vi "CurrentTrace.vi"() -> ()   [LabVIEW 2009]
uses:
  <vilib>/Utility/file.llb/Write To Spreadsheet File (DBL).vi
  <vilib>/express/express analysis/Spectral/XNode/ExpressSpectralMeasurementsBlockNode.xnode
  <vilib>/express/express analysis/Spectral/Block/exnSpectralBlock spectral measurements peak poly.vi
  <vilib>/express/express analysis/Spectral/Block/exnSpectralBlock spectral measurements peak DDT.vi
panel:
  in  "Enable":bool=TRUE
  in  "Filename":path=path "test.tdms"
  in  "String":string
  in  "Save Filtered Spectrum":bool
  in  "file path (use dialog) 4":path
  in  "Save Filtered Waveform":bool
  in  "file path (use dialog) 3":path
  in  "Save Unfiltered Spectrum":bool
  in  "file path (use dialog) 2":path
  in  "Save Unfiltered Waveform":bool
  in  "Boolean":bool
  in  "Bandpass Upper Cut-Off":dbl=313000.0 caption="Upper Cut-Off"
  in  "Bandpass Lower Cut-Off":dbl=312000.0 caption="Lower Cut-Off"
  in  "Low-Pass Cut-Off (Hz)":dbl=10000.0 caption="Lower Cut-Off"
  out "Filtered Spectrum":dynamicdata(graph)
  out "Unfiltered Spectrum":dynamicdata(graph)
  out "Filtered Signal":dynamicdata(graph)
  out "Unfiltered Signal":dynamicdata(graph)
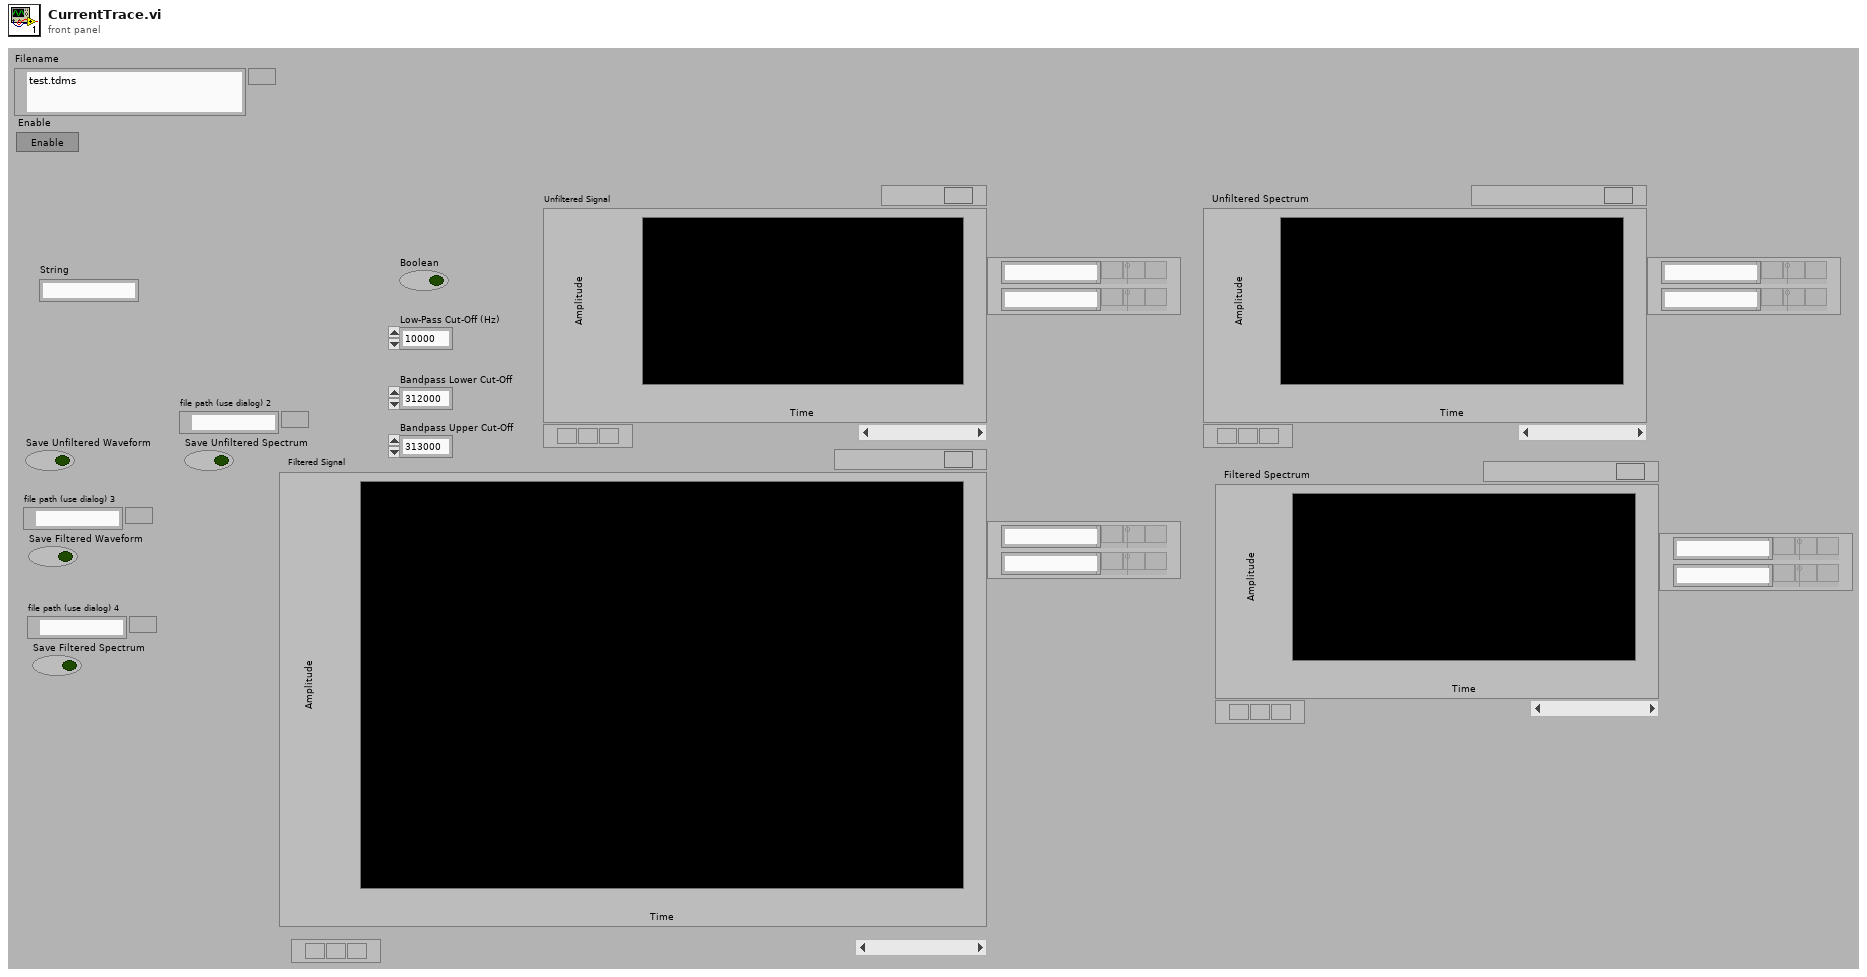
[diagram p1: front panel]
types:
  T1 = enum16{"open", "replace", "create", "open or create", "replace or create", "replace or create with confirmation"}
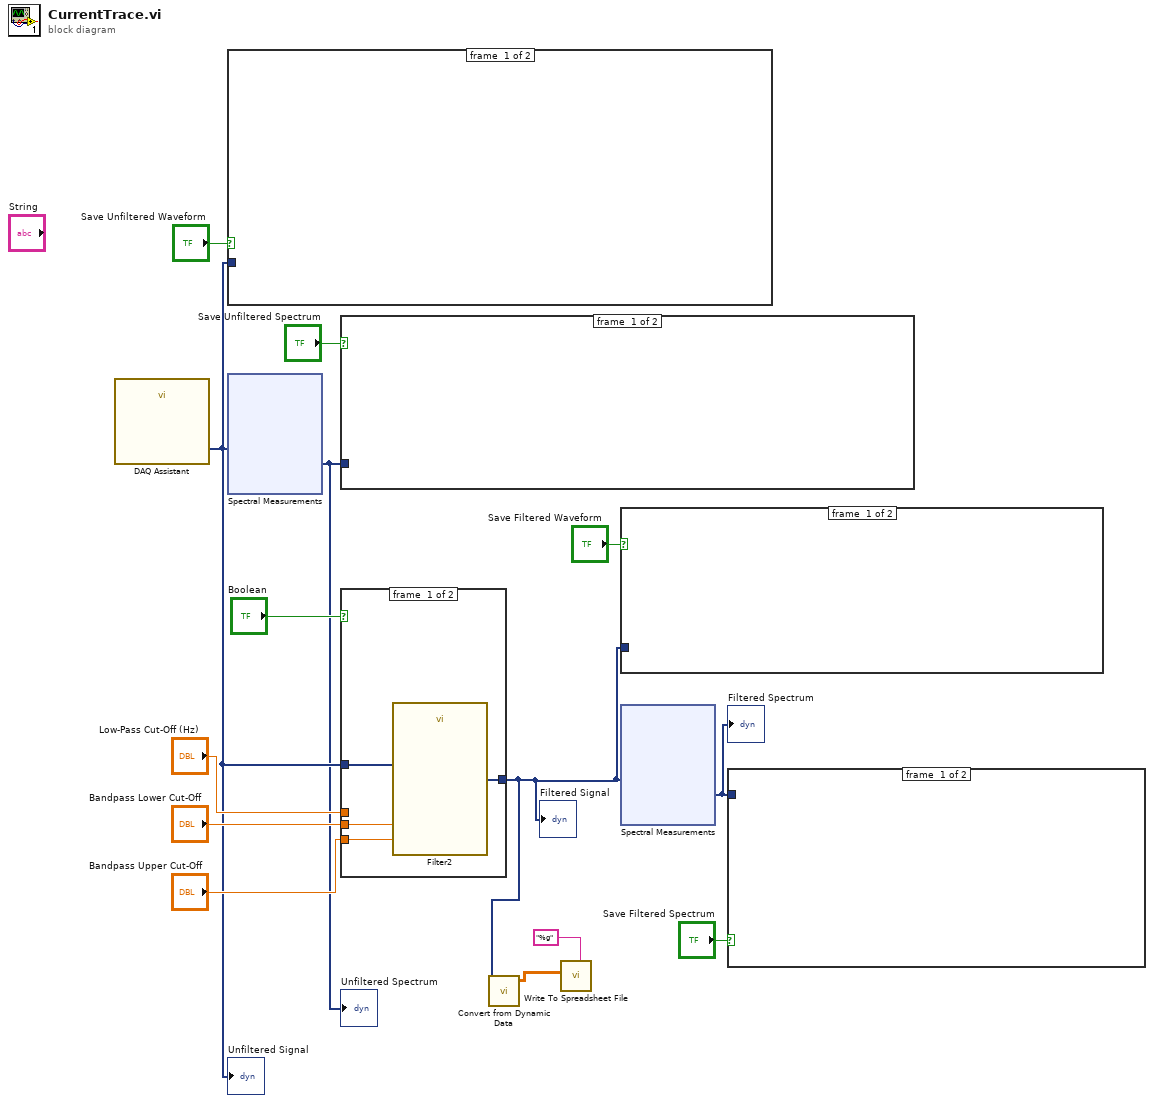
[diagram p0: block diagram]
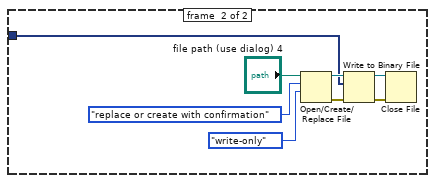
[diagram p2: hidden frame]
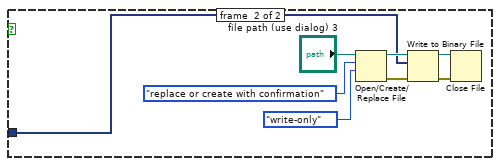
[diagram p3: hidden frame]
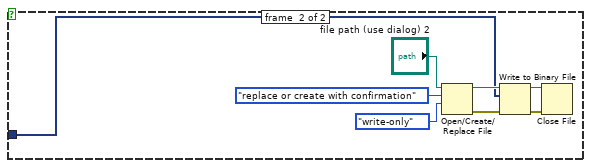
[diagram p4: hidden frame]
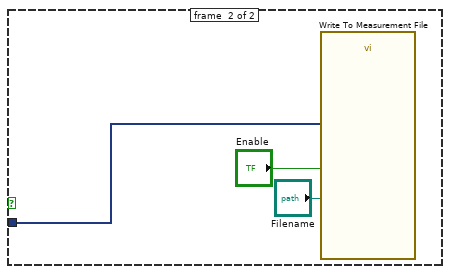
[diagram p5: hidden frame]
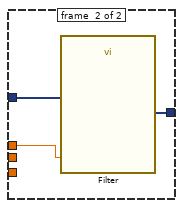
[diagram p6: hidden frame]
diagram:
  n1 = call "DAQ Assistant"() -> ("data"=w10:dynamicdata)  [unwired: 17 in, 2 out]
  "Unfiltered Signal" <- w10
  n2 = case shown="True" "Save Unfiltered Waveform" {
    tunnel: w10 -> [_ w17]
    frame #0 {
    }
    frame #1 {
      n3 = call "Write To Measurement File"("Signals"=w17, "Enable"="Enable", "Filename"="Filename") -> ()  [unwired: 14 in, 3 out]
    }
  }
  n4 = xnode "Spectral Measurements"("Signals"=w10) -> ("FFT - (Peak)"=w7:dynamicdata)  [unwired: 1 in, 2 out]
  "Unfiltered Spectrum" <- w7
  n5 = case shown="True" "Save Unfiltered Spectrum" {
    tunnel: w7 -> [_ w18]
    frame #0 {
    }
    frame #1 {
      n6 = Open/Create/Replace File(file path (use dialog)="file path (use dialog) 2", operation (0:open)=T1."replace or create with confirmation", access (0:read/write)=enum16{"read/write", "read-only", "write-only"}."write-only") -> (refnum out=w22:refnum<file>, error out=w21:errorcluster)  [unwired: 3 in, 1 out]
      n7 = Write to Binary File(file (use dialog)=w22, data=w18, error in=w21) -> (refnum out=w20:refnum<file>, error out=w19:errorcluster)  [unwired: 3 in, 1 out]
      n8 = Close File(refnum=w20, error in=w19) -> ()  [unwired: 2 out]
    }
  }
  n9 = case shown="True" "Boolean" {
    tunnel: "Low-Pass Cut-Off (Hz)" -> [_ w31]
    tunnel: "Bandpass Lower Cut-Off" -> [w29 _]
    tunnel: "Bandpass Upper Cut-Off" -> [w28 _]
    tunnel: w10 -> [w27 w32]
    tunnel: [w26 w30] -> w3
    frame #0 {
      n10 = call "Filter2"("Lower Cut-Off"=w29, "Upper Cut-Off"=w28, "Signal"=w27) -> ("Filtered Signal"=w26:dynamicdata)  [unwired: 7 in, 1 out]
    }
    frame #1 {
      n11 = call "Filter"("Lower Cut-Off"=w31, "Signal"=w32) -> ("Filtered Signal"=w30:dynamicdata)  [unwired: 8 in, 1 out]
    }
  }
  "Filtered Signal" <- w3
  n12 = call "Convert from Dynamic Data"("Dynamic Data Type"=w3) -> ("Array"=w1:dbl[][])  [unwired: 3 in]
  n13 = call-poly <vilib>:"Write To Spreadsheet File.vi"("format"="%g", "2D data"=w1) -> ()  [unwired: 6 in, 1 out]
  n14 = case shown="True" "Save Filtered Waveform" {
    tunnel: w3 -> [_ w33]
    frame #0 {
    }
    frame #1 {
      n15 = Open/Create/Replace File(file path (use dialog)="file path (use dialog) 3", operation (0:open)=T1."replace or create with confirmation", access (0:read/write)=enum16{"read/write", "read-only", "write-only"}."write-only") -> (refnum out=w37:refnum<file>, error out=w36:errorcluster)  [unwired: 3 in, 1 out]
      n16 = Write to Binary File(file (use dialog)=w37, data=w33, error in=w36) -> (refnum out=w35:refnum<file>, error out=w34:errorcluster)  [unwired: 3 in, 1 out]
      n17 = Close File(refnum=w35, error in=w34) -> ()  [unwired: 2 out]
    }
  }
  n18 = xnode "Spectral Measurements"("Signals"=w3) -> ("FFT - (Peak)"=w4:dynamicdata)  [unwired: 1 in, 2 out]
  "Filtered Spectrum" <- w4
  n19 = case shown="True" "Save Filtered Spectrum" {
    tunnel: w4 -> [_ w41]
    frame #0 {
    }
    frame #1 {
      n20 = Open/Create/Replace File(file path (use dialog)="file path (use dialog) 4", operation (0:open)=T1."replace or create with confirmation", access (0:read/write)=enum16{"read/write", "read-only", "write-only"}."write-only") -> (refnum out=w45:refnum<file>, error out=w44:errorcluster)  [unwired: 3 in, 1 out]
      n21 = Write to Binary File(file (use dialog)=w45, data=w41, error in=w44) -> (refnum out=w43:refnum<file>, error out=w42:errorcluster)  [unwired: 3 in, 1 out]
      n22 = Close File(refnum=w43, error in=w42) -> ()  [unwired: 2 out]
    }
  }
